vi "Laboratory_practice11.vi"() -> ()   [LabVIEW 2021]
panel:
  out "Waveform 1 Graph":dynamicdata(graph)
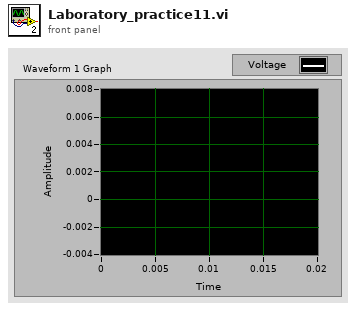
[diagram p1: front panel]
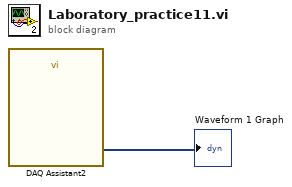
[diagram p0: block diagram]
diagram:
  n1 = call "DAQ Assistant2"() -> ("data"=→"Waveform 1 Graph":dynamicdata)  [unwired: 17 in, 2 out]
